vi "x-axis.vi"(8 "error in (no error)":errorcluster, 11 "Magna Voltage Scan in":refnum<class "Magna Voltage Scan.lvclass">) -> (0 "error out":errorcluster, 1 "Label":string, 2 "Unit":string, 3 "Magna Voltage Scan out":refnum<class "Magna Voltage Scan.lvclass">)   [LabVIEW 2015, in "Magna Voltage Scan.lvclass"]
uses:
  Magna Voltage Scan.lvclass
  Scanner/Scanner.lvclass
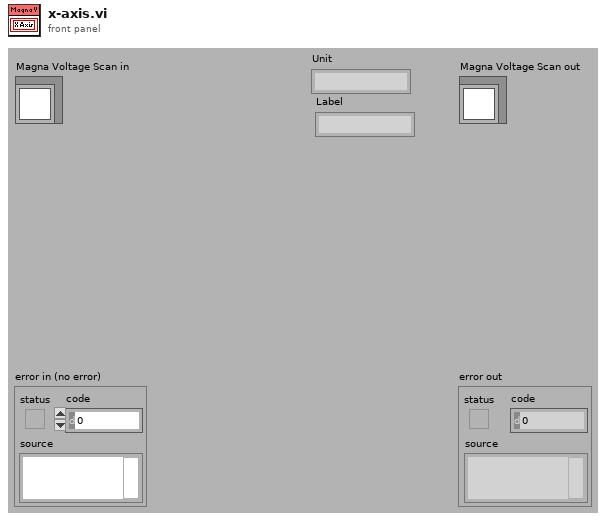
[diagram p1: front panel]
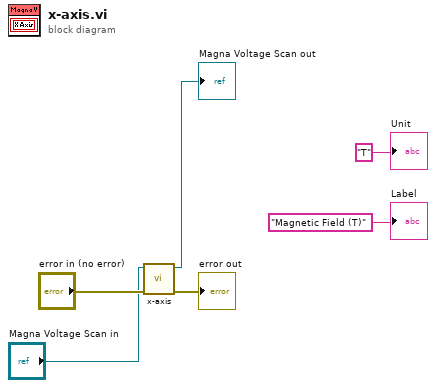
[diagram p0: block diagram]
diagram:
  n1 = call-parent "x-axis.vi"("error in (no error)"="error in (no error)", "Scanner in"="Magna Voltage Scan in") -> ("error out"=→"error out":errorcluster, "Scanner out"=→"Magna Voltage Scan out":refnum<class "Magna Voltage Scan.lvclass">)  [unwired: 6 in, 2 out]
  "Label" <- "Magnetic Field (T)" ("Label")
  "Unit" <- "T" ("Unit")
